vi "HP to kW.vi"(11 "Power (HP)":sgl) -> (3 "Power (kW)":i16)   [LabVIEW 2020]
doc: "Converts power from HP to kW.\n\nRounds single precision floating-point number to nearest integer and converts to 16-bit word integer."
panel:
  # "Power Conversion"
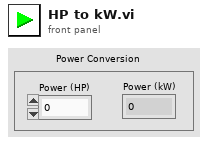
[diagram p1: front panel]
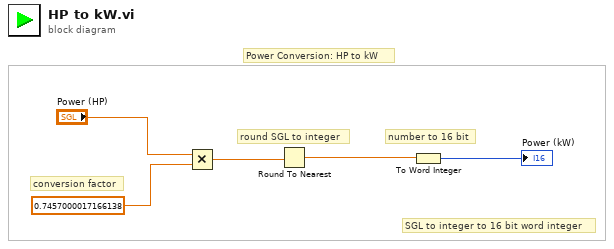
[diagram p0: block diagram]
diagram:
  # "Power Conversion: HP to kW"
  # "SGL to integer to 16 bit word integer"
  # "number to 16 bit"
  # "round SGL to integer"
  # "conversion factor"
  n1 = Multiply(x="Power (HP)", y=sgl 0.7457 ("x*y")) -> (x*y=w3:sgl)
  n2 = Round To Nearest(number=w3) -> (nearest integer value=w2:sgl)
  n3 = To Word Integer(number=w2) -> (16bit integer=→"Power (kW)":i16)
